vi "DHE_calcbuffers.vi"(4 "totpixelsin":u32, 7 "deftransferbufsize":u32=131072, 8 "error in (no error)":errorcluster, 9 "bpp":u8=16, 10 "nrows":u32, 11 "ncols":u32) -> (0 "virt buf bytes":u32, 1 "virt buf pixels":u32, 2 "Total image Bytes":u32, 3 "Total Pixels":u32, 6 "error out":errorcluster)   [LabVIEW 2016]
uses:
  DBSHAND/private/vis/DatabaseHand_Element_Get(string).vi
panel:
  out "phys buffers":i32
  out "remaining pixels":i32
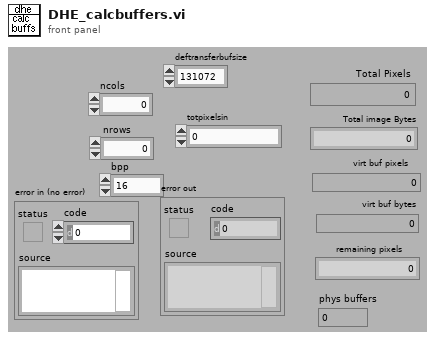
[diagram p1: front panel]
types:
  T1 = typedef "GEOM_Amplifier.ctl" = cluster{"number":i32, "type":T2, "rotated":i16, "fliped":u16, "FPAcoord":cluster{"xstart":i32, "ystart":i32}, "Physical_size":cluster{"columns":i32, "rows":i32}, "predata":cluster{"columns":i32, "rows":i32}, "postdata":cluster{"columns":i32, "rows":i32}, "Req ROIs":T3, "Corr ROI":T3, "Detnumber":i32, "ampID":string, "discard":i32}
  T2 = typedef "GEOM_AmpType.ctl" = u16
  T3 = typedef "GEOM_ROI.ctl" = T4[]
  T4 = typedef "GEOM_Coords.ctl" = cluster{"xstart":u32, "ystart":u32, "xsize":u32, "ysize":u32}
  T5 = typedef "CMN_Buffers.ctl" = cluster{"TotalPixels":u32, "Total image bytes":u32, "Total Phys Buffers":u32, "virtual buf pixels":u32, "virtual bytes size":u32, "Remaining piece":u32, "Transfer_Buf_size":u32}
  T6 = typedef "DatabaseHand_RefNum.ctl" = refnum<vi>
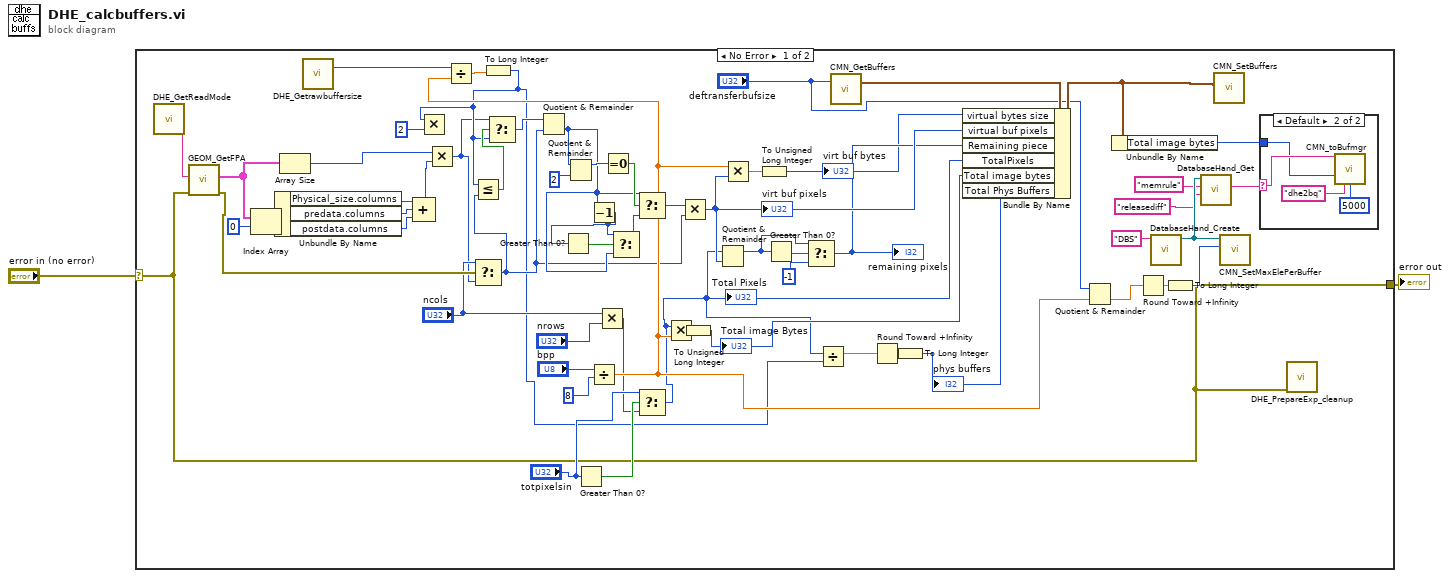
[diagram p0: block diagram]
diagram:
  n1 = case shown="No Error" "error in (no error)" {
    selector: "error in (no error)" -> [w21 w67]
    tunnel: [w21 w67] -> w1
    frame No Error {
      n2 = call "DHE_GetReadMode.vi"() -> ("DHE_ReadMode"=w22:string)  [unwired: 9 out]
      n3 = call "GEOM_GetFPA.vi"("error in (no error)"=w21, "readmode"=w22) -> ("error out"=w7:errorcluster, "amplifiers"=w17:T1[])  [unwired: 1 in, 7 out]
      n4 = Index Array(array=w17, index=0) -> (element=w19:T1)
      n5 = Unbundle By Name(w19) -> ("Physical_size.columns"=w16:i32, "predata.columns"=w15:i32, "postdata.columns"=w14:i32)
      n6 = Array Size(array=w17) -> (size(s)=w18:i32)
      n7 = call "DHE_Getrawbuffersize.vi"() -> ("DHE_raw_buffer_size"=w12:i32)  [unwired: 9 out]
      n8 = Compound Arithmetic op=ADD(w16, w15, w14) -> (w13:i32)
      n9 = Multiply(x=w18, y=w13) -> (x*y=w3:i32)
      n10 = Select(t="ncols", s=w7, f=w3) -> (s? t:f=w11:u32)
      n11 = Greater Than 0?(x="totpixelsin") -> (x > 0?=w38:bool)
      n12 = Divide(x="bpp", y=8) -> (x/y=w42:dbl)
      n13 = Divide(x=w12, y=w42) -> (x/y=w45:dbl)
      n14 = To Long Integer(number=w45) -> (32bit integer=w4:i32)
      n15 = Multiply(x=w4, y=2) -> ()  [unwired: 1 out]
      n16 = Less Or Equal?(x=w4, y=w11) -> (x <= y?=w5:bool)
      n17 = Select(t=w3, s=w5, f=w4) -> (s? t:f=w10:i32)
      n18 = Quotient & Remainder(x=w10, y=w11) -> (floor(x/y)=w23:u32)  [unwired: 1 out]
      n19 = Quotient & Remainder(x=w23, y=2) -> (x-y*floor(x/y)=w61:u32)  [unwired: 1 out]
      n20 = Decrement(x=w23) -> (x-1=w25:u32)
      n21 = Greater Than 0?(x=w25) -> (x > 0?=w26:bool)
      n22 = Multiply(x="ncols", y="nrows") -> (x*y=w36:u32)
      n23 = Equal To 0?(x=w61) -> (x = 0?=w34:bool)
      n24 = Select(t=w25, s=w26, f=w23) -> (s? t:f=w24:u32)
      n25 = Select(t=w23, s=w34, f=w24) -> (s? t:f=w60:u32)
      n26 = Select(t="totpixelsin", s=w38, f=w36) -> (s? t:f=w35:u32)
      "Total Pixels" <- w35
      n27 = Multiply(x=w35, y=w42) -> (x*y=w56:dbl)
      n28 = Multiply(x=w60, y=w11) -> (x*y=w54:u32)
      "virt buf pixels" <- w54
      n29 = To Unsigned Long Integer(number=w56) -> (unsigned 32bit integer=w47:u32)
      "Total image Bytes" <- w47
      n30 = Quotient & Remainder(x=w35, y=w54) -> (x-y*floor(x/y)=w58:u32)  [unwired: 1 out]
      n31 = Multiply(x=w42, y=w54) -> (x*y=w49:dbl)
      n32 = To Unsigned Long Integer(number=w49) -> (unsigned 32bit integer=w48:u32)
      "virt buf bytes" <- w48
      n33 = Greater Than 0?(x=w58) -> (x > 0?=w59:bool)
      n34 = Select(t=w58, s=w59, f=-1) -> (s? t:f=w53:u32)
      "remaining pixels" <- w53
      n35 = Divide(x=w35, y=w4) -> (x/y=w52:dbl)
      n36 = call "CMN_GetBuffers.vi"("deftransferbufsize"="deftransferbufsize") -> ("BuffersDimensions"=w44:T5)  [unwired: 1 in, 9 out]
      n37 = Round Toward +Infinity(x=w52) -> (ceil(x): smallest int >= x=w51:dbl)
      n38 = To Long Integer(number=w51) -> (32bit integer=w46:i32)
      "phys buffers" <- w46
      n39 = Bundle By Name(cluster=w44, "virtual bytes size"=w48, "virtual buf pixels"=w54, "Remaining piece"=w53, "TotalPixels"=w35, "Total image bytes"=w47, "Total Phys Buffers"=w46) -> (w28:T5)
      n40 = Quotient & Remainder(x="deftransferbufsize", y=w42) -> (floor(x/y)=w41:dbl)  [unwired: 1 out]
      n41 = Unbundle By Name(w28) -> ("Total image bytes"=w27:u32)
      n42 = Round Toward +Infinity(x=w41) -> (ceil(x): smallest int >= x=w40:dbl)
      n43 = call "DatabaseHand_Create.vi"("Name"="DBS") -> ("Database RefNum out"=w32:T6)  [unwired: 1 in, 9 out]
      n44 = To Long Integer(number=w40) -> (32bit integer=w39:i32)
      n45 = call-poly "DatabaseHand_Get.vi"("default value"="releasediff", "name"="memrule", "Database RefNum in"=w32) -> ("value"=w29:string)  [unwired: 2 in, 6 out]
      n46 = call "CMN_SetBuffers.vi"("BuffersDimensions"=w28) -> ()  [unwired: 2 in, 9 out]
      n47 = call "CMN_SetMaxElePerBuffer.vi"("maxele_per_read_buffer"=w39, "Database RefNum"=w32) -> ()  [unwired: 10 out]
      n48 = case shown="Default" w29 {
        selector: w29 -> [_ w64]
        tunnel: w27 -> [_ w63]
        frame "", "false", "no", "none", "off" {
        }
        frame Default {
          n49 = call "CMN_toBufmgr.vi"("command"=w64, "bufsize"=w63, "responseQ"="dhe2bq", "ms timeout (-1)"=5000) -> ()  [unwired: 4 in, 8 out]
        }
      }
      n50 = call "DHE_PrepareExp_cleanup.vi"("error in (no error)"=w21) -> ()  [unwired: 11 out]
    }
    frame Error {
    }
  }
  "error out" <- w1
